vi "Drag Ended.vi"(8 "error in (no error)":errorcluster, 11 "BetterBoxHandle in":refnum<class "BetterBoxHandle.lvclass">) -> (0 "error out":errorcluster, 3 "BetterBoxHandle out":refnum<class "BetterBoxHandle.lvclass">)   [LabVIEW 2020, in "BetterDragAndDrop.lvlib" / "BetterBoxHandle.lvclass"]
uses:
  BetterBoxHandle.lvclass
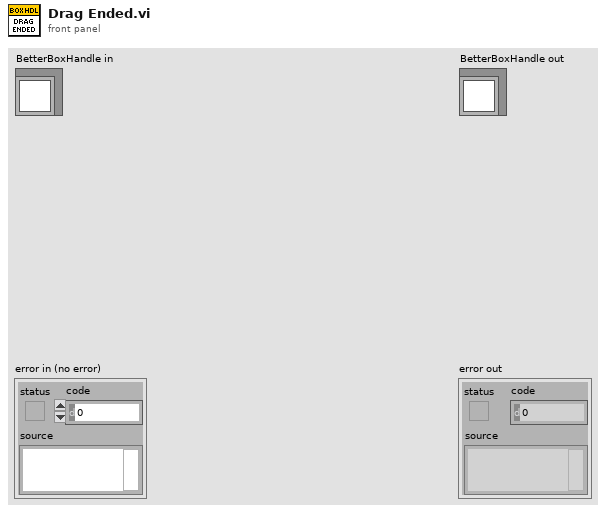
[diagram p1: front panel]
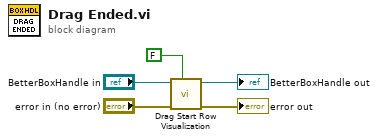
[diagram p0: block diagram]
diagram:
  n1 = call-dynamic "Drag Start Row Visualization.vi"("DragStart? (F)"=FALSE, "error in (no error)"="error in (no error)", "BetterBoxHandle in"="BetterBoxHandle in") -> ("error out"=→"error out":errorcluster, "BetterBoxHandle out"=→"BetterBoxHandle out":refnum<class "BetterBoxHandle.lvclass">)  [unwired: 7 in]
